vi "Read Step Data (AC Polyphase Total Program Mode).vi"(0 "VISA resource name":refnum<visa-resource-name>, 5 "Step (1)":i32=1 min=1 max=9 format="%2_0f", 11 "error in (no error)":errorcluster) -> (4 "VISA resource name out":refnum<visa-resource-name>, 6 "Test Meter Data Output":T1 {"Timer (s)" format="%.1f"}, 15 "error out":errorcluster)   [LabVIEW 2016, in "APT 300XAC Series.lvlib"]
doc: "Reads the Program mode <B>result data for phase B</B> while the test has ended.\n\nIn Program Mode the output data cluster has the following data.\n\n1. Memory\n2. Step\n3. Timer (s)\n4. Frequency (Hz)\n5. Voltage (V)\n6. RMS Current (A)\n7. Power (W)\n8. Peak Current (A)\n9. Power Factor\n10. Status\n11. Power Resistive (VAR)\n12. Crest Factor\n13. Power Apparent (VA)"
uses:
  APT 300XAC Series.lvlib
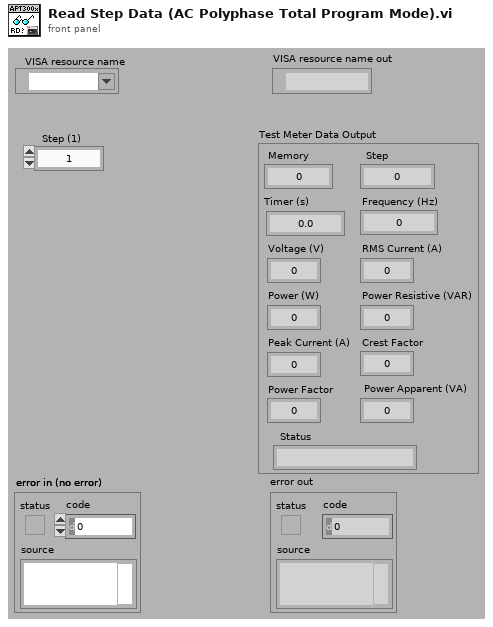
[diagram p1: front panel]
types:
  T1 = cluster{"Memory":i32, "Step":i32, "Timer (s)":dbl, "Frequency (Hz)":dbl, "Voltage (V)":dbl, "RMS Current (A)":dbl, "Power (W)":dbl, "Peak Current (A)":dbl, "Power Factor":dbl, "Status":string, "Power Resistive (VAR)":dbl, "Crest Factor":dbl, "Power Apparent (VA)":dbl}
  T2 = cluster{"Memory":i32, "Step":i32, "Timer":dbl, "Frequency":dbl, "Volt":dbl, "Current":dbl, "Power":dbl, "Peak Current":dbl, "Power Factor":dbl, "Status":string, "Power Resistive":dbl, "Crest Factor":dbl, "Power Apparent":dbl}
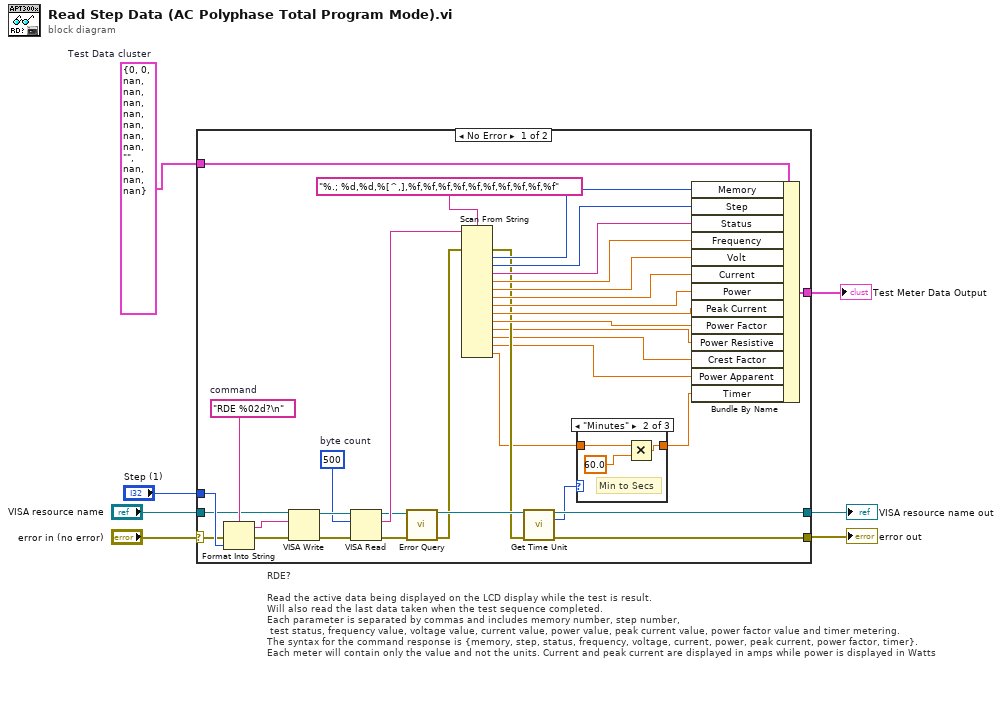
[diagram p0: block diagram]
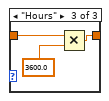
[diagram p3: hidden frame]
diagram:
  w3 = T2 {"Memory"=0, "Step"=0, "Timer"=nan, "Frequency"=nan, "Volt"=nan, "Current"=nan, "Power"=nan, "Peak Current"=nan, "Power Factor"=nan, "Status"="", "Power Resistive"=nan, "Crest Factor"=nan, "Power Apparent"=nan}  # Test Data cluster
  # "RDE?\n\nRead the active data being displayed on the LCD display while the test is result. \nWill also read the last data taken when the test sequence completed. \nEach parameter is separated by commas and includes memory number, step number,\n test status, frequency value, voltage value, current value, power value, peak current value, power factor value and timer metering. \nThe syntax for the command response is {memory, step, status, frequency, voltage, current, power, peak current, power factor, timer}. \nEach meter will contain only the value and not the units. Current and peak current are displayed in amps while power is displayed in Watts"
  n1 = case shown="No Error" "error in (no error)" {
    selector: "error in (no error)" -> [w11 w51]
    tunnel: "VISA resource name" -> [w9 w52]
    tunnel: [w36 w52] -> w5
    tunnel: [w37 w51] -> w4
    tunnel: [w39 w50] -> w2
    tunnel: w3 -> [w38 w50]
    tunnel: "Step (1)" -> [w12 _]
    frame No Error {
      w13 = "RDE %02d?\n"  # command
      w40 = u32 500  # byte count
      n2 = Format Into String(format string=w13, error in=w11, w12) -> (resulting string=w8:string, error out=w10:errorcluster)  [unwired: 1 in]
      n3 = VISA Write(VISA resource name=w9, write buffer=w8, error in (no error)=w10) -> (VISA resource name out=w42:refnum<visa-resource-name>, error out=w41:errorcluster)  [unwired: 1 out]
      n4 = VISA Read(VISA resource name=w42, byte count=w40, error in (no error)=w41) -> (VISA resource name out=w23:refnum<visa-resource-name>, read buffer=w24:string, error out=w22:errorcluster)  [unwired: 1 out]
      n5 = call "Error Query.vi"("VISA resource name"=w23, "error in (no error)"=w22) -> ("VISA resource name out"=w21:refnum<visa-resource-name>, "error out"=w20:errorcluster)  [unwired: 10 in, 2 out]
      n6 = Scan From String(format string="%.; %d,%d,%[^,],%f,%f,%f,%f,%f,%f,%f,%f,%f,%f", input string=w24, error in=w20) -> (error out=w19:errorcluster, output 1=w33:i32, output 2=w32:i32, output 3=w31:string, output 4=w30:dbl, output 5=w29:dbl, output 6=w28:dbl, output 7=w27:dbl, output 8=w26:dbl, output 9=w25:dbl, output 10=w17:dbl, output 11=w16:dbl, output 12=w15:dbl, output 13=w18:dbl)  [unwired: 14 in, 2 out]
      n7 = call "Get Time Unit.vi"("VISA resource name"=w21, "error in (no error)"=w19) -> ("VISA resource name out"=w36:refnum<visa-resource-name>, "Time Unit"=w35:enum16{"Seconds", "Minutes", "Hours"}, "error out"=w37:errorcluster)  [unwired: 11 in]
      n8 = case shown="\"Minutes\"" w35 {
        tunnel: [w43 w45 w48] -> w14
        tunnel: w18 -> [w43 w44 w47]
        frame "Seconds" {
        }
        frame "Minutes" {
          # "Min to Secs"
          n9 = Multiply(x=w44, y=60.0) -> (x*y=w45:dbl)
        }
        frame "Hours" {
          n10 = Multiply(x=w47, y=3600.0) -> (x*y=w48:dbl)
        }
      }
      n11 = Bundle By Name(cluster=w38, "Memory"=w33, "Step"=w32, "Status"=w31, "Frequency"=w30, "Volt"=w29, "Current"=w28, "Power"=w27, "Peak Current"=w26, "Power Factor"=w25, "Power Resistive"=w17, "Crest Factor"=w16, "Power Apparent"=w15, "Timer"=w14) -> (w39:T2)
    }
    frame Error {
    }
  }
  "VISA resource name out" <- w5
  "error out" <- w4
  "Test Meter Data Output" <- w2
